vi "Insert XML node.vi"(8 "error in":errorcluster, 9 "Text":string, 10 "Tag":string) -> (0 "error out":errorcluster, 3 "XML text":string)   [LabVIEW 2013]
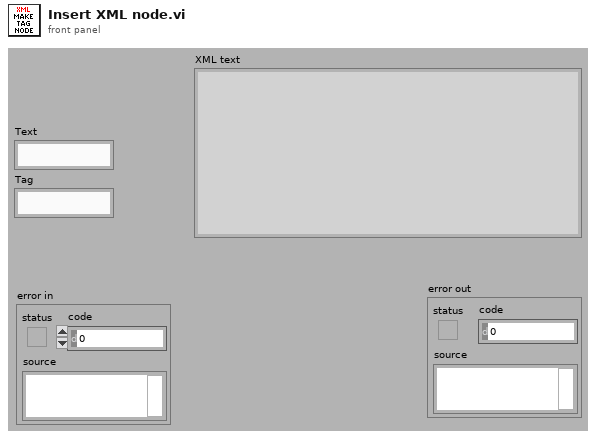
[diagram p1: front panel]
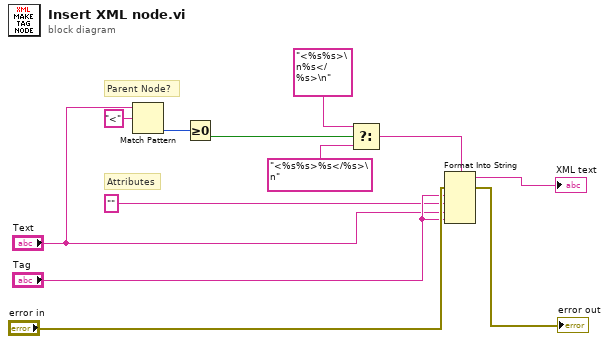
[diagram p0: block diagram]
diagram:
  # "Parent Node?"
  # "Attributes"
  n1 = Match Pattern(string="Text", regular expression="<") -> (offset past match=w4:i32)  [unwired: 1 in, 3 out]
  n2 = Greater Or Equal To 0?(x=w4) -> (x >= 0?=w1:bool)
  n3 = Select(t="<%s%s>\n%s</%s>\n" ("format string"), s=w1, f="<%s%s>%s</%s>\n" ("format string")) -> (s? t:f=w10:string)
  n4 = Format Into String(format string=w10, error in="error in", "Tag", "" ("input 2"), "Text", "Tag") -> (resulting string=→"XML text":string, error out=→"error out":errorcluster)  [unwired: 1 in]
